vi "CheckForExistingFITS.vi"(0 "Filename":string, 1 "error in":errorcluster) -> (2 "New Filename":string, 3 "New Exposure #":i32 format="%04.0f", 4 "error out":errorcluster)   [LabVIEW 2015]
uses:
  Instance           1 28Saved   CheckForExistingFITS .vi
panel:
  out "code":i32
  out "path":path
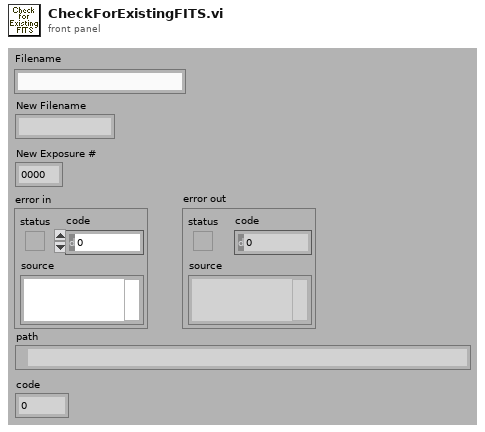
[diagram p1: front panel]
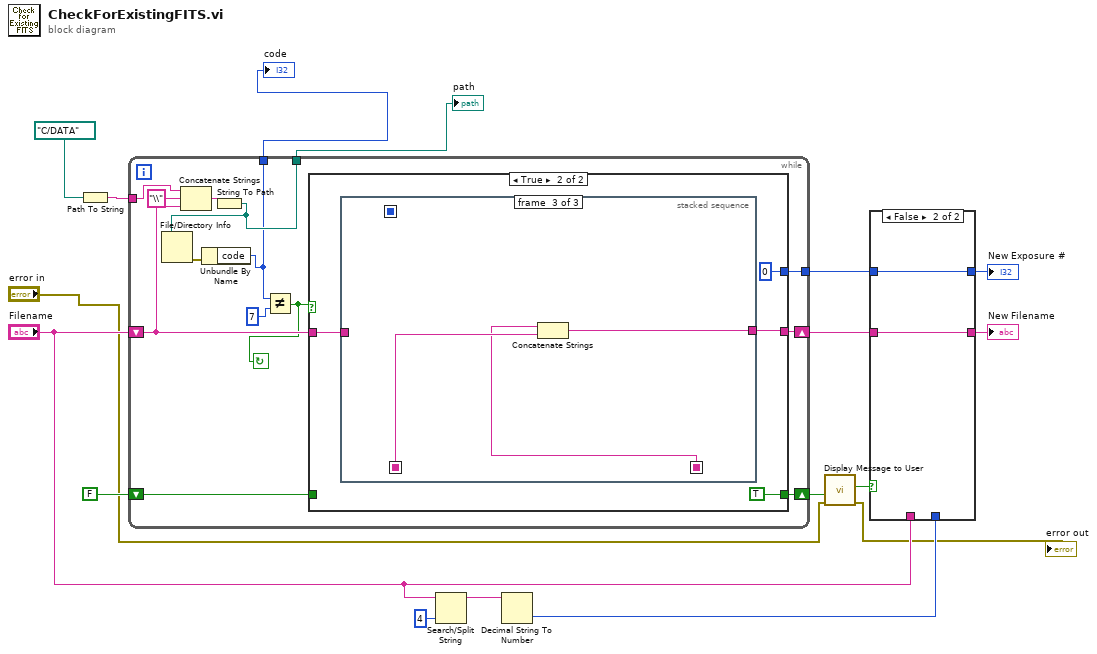
[diagram p0: block diagram]
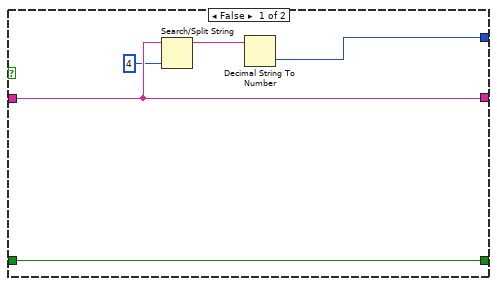
[diagram p3: hidden frame]
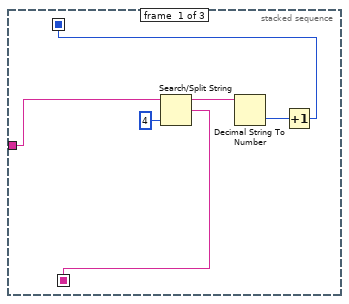
[diagram p4: hidden frame]
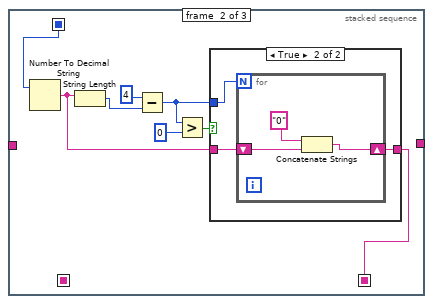
[diagram p5: hidden frame]
diagram:
  n1 = Path To String(path=path "C:/DATA" ("directory path")) -> (string=w4:string)
  n2 = while {
    shift-right: [w30] -> w15
    shift-left: "Filename" -> [w26]
    tunnel: [w29] -> w16
    shift-right: [w28] -> w8
    shift-left: FALSE -> [w27]
    tunnel: w4 -> [w23]
    tunnel: [w21] -> w2
    tunnel: [w18] -> w1
    stop <- w19 continue-if-true
    n3 = Concatenate Strings(w23, "\\" ("string"), w26) -> (w25:string)
    n4 = String To Path(string=w25) -> (path=w21:path)
    n5 = File/Directory Info(path=w21) -> (error out=w24:errorcluster)  [unwired: 1 in, 6 out]
    n6 = Unbundle By Name(w24) -> ("code"=w18:i32)
    n7 = Not Equal?(x=w18, y=7) -> (x != y?=w19:bool)
    n8 = case shown="True" w19 {
      tunnel: [w35 w39] -> w30
      tunnel: w26 -> [w35 w36]
      tunnel: [w32 0 ("offset past number")] -> w29
      tunnel: [w31 TRUE] -> w28
      tunnel: w27 -> [w31 _]
      frame False {
        n9 = Search/Split String(string=w35, offset (0)=4) -> (substring before match=w33:string)  [unwired: 1 in, 2 out]
        n10 = Decimal String To Number(string=w33) -> (number=w32:i32)  [unwired: 2 in, 1 out]
      }
      frame True {
        n11 = stacked-sequence {
          seq-local: [w42 _ _] -> [_ _ w63]
          seq-local: [w41 _ _] -> [_ w53 _]
          seq-local: [_ w46 _] -> [_ _ w61]
          tunnel: [_ _ w62] -> w39
          tunnel: w36 -> [w40 _ _]
          frame #0 {
            n12 = Search/Split String(string=w40, offset (0)=4) -> (substring before match=w44:string, match + rest of string=w42:string)  [unwired: 1 in, 1 out]
            n13 = Decimal String To Number(string=w44) -> (number=w43:i32)  [unwired: 2 in, 1 out]
            n14 = Increment(x=w43) -> (x+1=w41:i32)
          }
          frame #1 {
            n15 = Number To Decimal String(number=w53) -> (decimal integer string=w47:string)  [unwired: 1 in]
            n16 = String Length(string=w47) -> (length=w52:i32)
            n17 = Subtract(x=4 ("y"), y=w52) -> (x-y=w48:i32)
            n18 = Greater?(x=w48, y=0) -> (0:w49:bool)
            n19 = case shown="True" w49 {
              tunnel: w48 -> [_ w57]
              tunnel: w47 -> [w54 w56]
              tunnel: [w54 w55] -> w46
              frame False {
              }
              frame True {
                n20 = for {
                  N: w57 -> [_]
                  shift-right: [w58] -> w55
                  shift-left: w56 -> [w60]
                  n21 = Concatenate Strings("0" ("string"), w60) -> (w58:string)
                }
              }
            }
          }
          frame #2 {
            n22 = Concatenate Strings(w61, w63) -> (w62:string)
          }
        }
      }
    }
  }
  "path" <- w2
  "code" <- w1
  n23 = Search/Split String(string="Filename", offset (0)=4) -> (substring before match=w10:string)  [unwired: 1 in, 2 out]
  n24 = Decimal String To Number(string=w10) -> (number=w9:i32)  [unwired: 2 in, 1 out]
  n25 = call "Display Message to User"("error in (no error)"="error in", "Enable"=w8) -> ("error out"=→"error out":errorcluster, "Yes"=w7:bool)  [unwired: 8 in]
  n26 = case shown="False" w7 {
    tunnel: w16 -> [_ w66]
    tunnel: w15 -> [_ w67]
    tunnel: [w64 w67] -> w14
    tunnel: [w65 w66] -> w13
    tunnel: "Filename" -> [w64 _]
    tunnel: w9 -> [w65 _]
    frame True {
    }
    frame False {
    }
  }
  "New Filename" <- w14
  "New Exposure #" <- w13
